vi "GetIMUAverage.vi"(0 "ADI IMU Interrupt DevRef In":T1={"ADI IMU DevRef"={"DevStatus"={"status"=FALSE, "code"=0, "source"=""}, "Handle"=0, "SPI Bus"=enum."SPI On-Board, CS0", "Device Found"=FALSE, "Device Ready"=FALSE, "Yaw Axis"=enum."Z", "AHRS Algorithm"=enum."Complementary", "Serial"=0, "Lot ID 2"=0, "Lot ID 1"=0, "Product ID"=0}, "InterruptRef"={"DevStatus"={"status"=FALSE, "code"=0, "source"=""}, "InterruptIndex"=enum."0"}}, 1 "error in":errorcluster) -> (2 "ADI IMU Interrupt DevRef Out":T1={"ADI IMU DevRef"={"DevStatus"={"status"=FALSE, "code"=0, "source"=""}, "Handle"=0, "SPI Bus"=enum."SPI On-Board, CS0", "Device Found"=FALSE, "Device Ready"=FALSE, "Yaw Axis"=enum."Z", "AHRS Algorithm"=enum."Complementary", "Serial"=0, "Lot ID 2"=0, "Lot ID 1"=0, "Product ID"=0}, "InterruptRef"={"DevStatus"={"status"=FALSE, "code"=0, "source"=""}, "InterruptIndex"=enum."0"}}, 3 "mean":dbl format="%0.2f", 4 "error out":errorcluster)   [LabVIEW 2016]
uses:
  <vilib>/Rock Robotics/WPI/ThirdParty/Sensors/ADIS16448 IMU/ADI_IMU_ADIS16448_InterruptDevRef.ctl
  <vilib>/Rock Robotics/WPI/ThirdParty/Sensors/ADIS16448 IMU/ADI_IMU_ADIS16448_IMUDevRef.ctl
  <vilib>/Rock Robotics/SystemInterfaces/spilib/spi_bus.ctl
  <vilib>/Rock Robotics/WPI/Interrupt/WPI_InterruptRef.ctl
  <vilib>/Rock Robotics/SystemInterfaces/Interrupt/FPGA_InterruptIndex.ctl
  <vilib>/Analysis/baseanly.llb/Mean (DBL).vi
  <vilib>/Analysis/NI_AALBase.lvlib
  <vilib>/Rock Robotics/WPI/ThirdParty/Sensors/ADIS16448 IMU/ADIS16448_IMU.lvlib
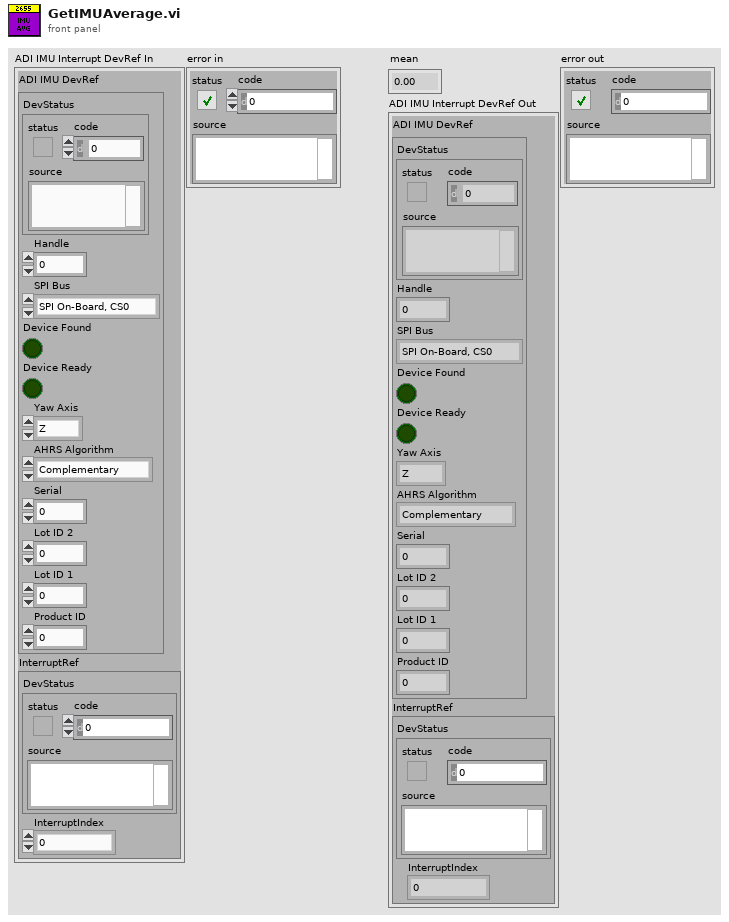
[diagram p1: front panel]
types:
  T1 = typedef "ADIS16448_IMU.lvlib/ADI_IMU_ADIS16448_InterruptDevRef.ctl" = cluster{"ADI IMU DevRef":T2, "InterruptRef":T4}
  T2 = typedef "ADIS16448_IMU.lvlib/ADI_IMU_ADIS16448_IMUDevRef.ctl" = cluster{"DevStatus":errorcluster, "Handle":i32, "SPI Bus":T3, "Device Found":bool, "Device Ready":bool, "Yaw Axis":enum16{"X", "Y", "Z"}, "AHRS Algorithm":enum16{"Complementary", "Madgwick"}, "Serial":u16, "Lot ID 2":u16, "Lot ID 1":u16, "Product ID":u16}
  T3 = typedef "spi_bus.ctl" = enum16{"SPI On-Board, CS0", "SPI On-Board, CS1", "SPI On-Board, CS2", "SPI On-Board, CS3", "SPI MXP", "Invalid"}
  T4 = typedef "WPI_InterruptRef.ctl" = cluster{"DevStatus":errorcluster, "InterruptIndex":T5}
  T5 = typedef "FPGA_InterruptIndex.ctl" = enum8{"0", "1", "2", "3", "4", "5", "6", "7", "Invalid"}
  T6 = cluster{"X Angle":dbl, "Y Angle":dbl, "Z Angle":dbl}
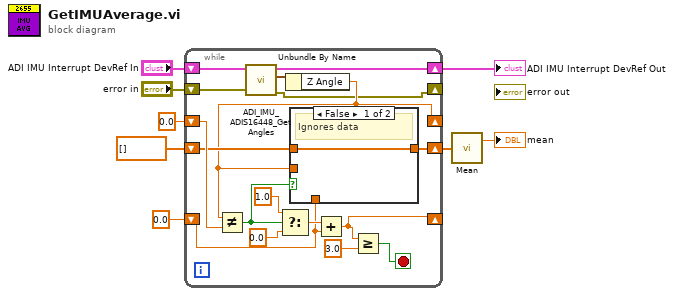
[diagram p0: block diagram]
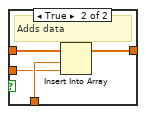
[diagram p2: hidden frame]
diagram:
  n1 = while {
    shift-right: [w16] -> _
    shift-left: 0.0 ("Z Angle") -> [w25]
    shift-right: [w17] -> _
    shift-left: 0.0 -> [w14]
    shift-right: [w12] -> w3
    shift-left: "ADI IMU Interrupt DevRef In" -> [w11]
    shift-right: [w15] -> w7
    shift-left: dbl[] [] -> [w18]
    shift-right: [w9] -> _
    shift-left: "error in" -> [w10]
    stop <- w21 stop-if-true
    n2 = call <vilib>:"ADI_IMU_ADIS16448_Get Angles.vi"("error in"=w10, "ADI IMU Interrupt DevRef"=w11) -> ("error out"=w9:errorcluster, "IMU Angles Out"=w13:T6, "ADI IMU Interrupt DevRef Out"=w12:T1)  [unwired: 6 in, 1 out]
    n3 = Unbundle By Name(w13) -> ("Z Angle"=w16:dbl)
    n4 = Not Equal?(x=w16, y=w25) -> (x != y?=w19:bool)
    n5 = Select(t=1.0, s=w19, f=0.0) -> (s? t:f=w22:dbl)
    n6 = case shown="False" w19 {
      tunnel: w18 -> [w26 w30]
      tunnel: [w26 w29] -> w15
      tunnel: w16 -> [_ w27]
      tunnel: w14 -> [_ w28]
      frame False {
        # "Ignores data"
      }
      frame True {
        # "Adds data"
        n7 = Insert Into Array(array=w30, index=w28, new element=w27) -> (w29:dbl[])
      }
    }
    n8 = Add(x=w22, y=w14) -> (x+y=w17:dbl)
    n9 = Greater Or Equal?(x=w17, y=3.0) -> (x >= y?=w21:bool)
  }
  "ADI IMU Interrupt DevRef Out" <- w3
  n10 = call-poly <vilib>:"Mean.vi"("X"=w7) -> ("mean"=→"mean":dbl)  [unwired: 1 out]
